vi "DSF.Engine.Plugin.Initialize.vi"(8 "error in (no error)":errorcluster, 10 "Cache":refnum<class "DSF.Engine.Memory.Cache.lvclass">, 11 "Plugin in":refnum<class "DSF.Engine.Plugin.lvclass">) -> (0 "error out":errorcluster, 3 "Plugin out":refnum<class "DSF.Engine.Plugin.lvclass">)   [LabVIEW 2017, in "DSF.Engine.lvlib" / "DSF.Engine.Plugin.lvclass"]
uses:
  DSF.Engine.Plugin.lvclass
  Cache/DSF.Engine.Memory.Cache.lvclass
  DSF.Engine.Plugin.lvclass/DSF.Engine.Plugin.ctl
  Timing/DSF.Engine.Timing.lvclass/DSF.Engine.Timing.ctl
  Debug/DSF.Engine.Debug Flags.lvclass/DSF.Engine.Debug Flags.ctl
  Thread Pool/DSF.Engine.Pool.lvclass/DSF.Engine.Pool.ctl
  Debug/DSF.Engine.Debug Flags.FIFO.lvclass/DSF.Engine.Debug Flags.FIFO.ctl
  Thread Pool/DSF.Engine.Pool.Read FIFO.vi
  Thread Pool/DSF.Engine.Pool.Write FIFO.vi
  Thread Pool/DSF.Engine.Pool.Get FIFO.vi
  Thread Pool/DSF.Engine.Pool.Get Debug Flags.vi
  Debug/DSF.Engine.Debug Flags.FIFO.Get Infinite Timeouts.vi
  Thread Pool/DSF.Engine.Pool.ID.lvclass
  C:/Git/DSF/Source/Engine/Classes/Thread Pool/DSF.Engine.Pool.lvclass
  Transceiver/DSF.Engine.Transceiver Thread.lvclass
  Thread Parameters/Thread Parameters.lvclass
  Timing/DSF.Engine.Timing.lvclass
  Debug/DSF.Engine.Debug Flags.lvclass
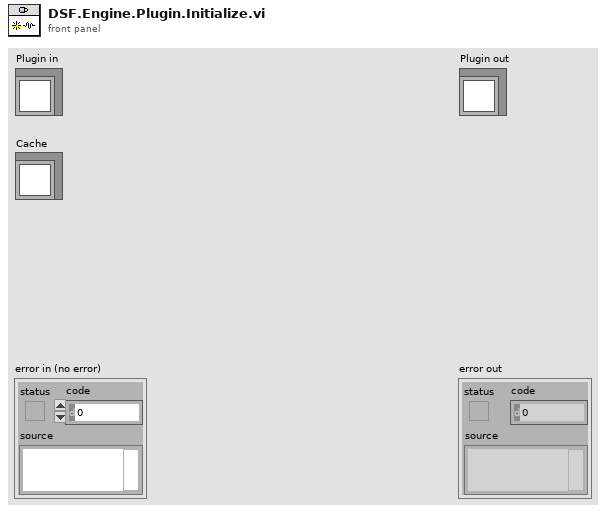
[diagram p1: front panel]
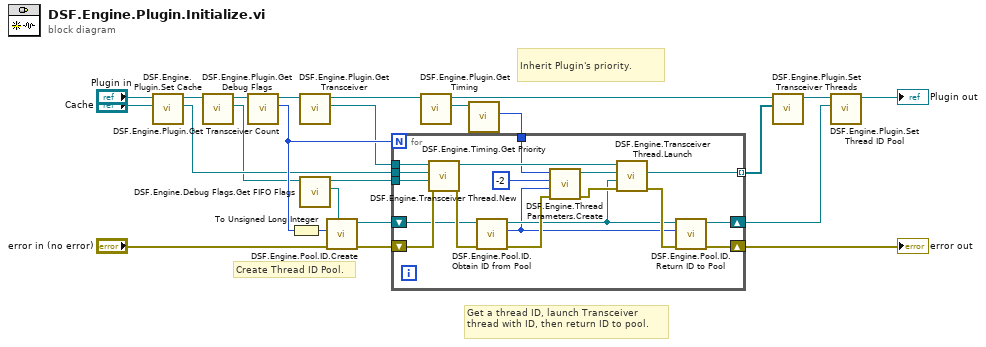
[diagram p0: block diagram]
diagram:
  # "Inherit Plugin's priority."
  # "Get a thread ID, launch Transceiver thread with ID, then return ID to pool."
  # "Create Thread ID Pool."
  n1 = call "DSF.Engine.Plugin.Set Cache.vi"("Cache"="Cache", "Plugin in"="Plugin in") -> ("Plugin out"=w7:refnum<class "DSF.Engine.Plugin.lvclass">)  [unwired: 9 in]
  n2 = call "DSF.Engine.Plugin.Get Debug Flags.vi"("Plugin in"=w7) -> ("Debug Flags"=w4:refnum<class "DSF.Engine.Debug Flags.lvclass">, "Plugin out"=w6:refnum<class "DSF.Engine.Plugin.lvclass">)  [unwired: 9 in]
  n3 = call "DSF.Engine.Plugin.Get Transceiver Count.vi"("Plugin in"=w6) -> ("transceiver count"=w14:i32, "Plugin out"=w19:refnum<class "DSF.Engine.Plugin.lvclass">)  [unwired: 9 in]
  n4 = To Unsigned Long Integer(number=w14) -> (unsigned 32bit integer=w15:u32)
  n5 = call "DSF.Engine.Plugin.Get Transceiver.vi"("Plugin in"=w19) -> ("Transceiver"=w2:refnum<class "DSF.Engine.Transceiver.lvclass">, "Plugin out"=w23:refnum<class "DSF.Engine.Plugin.lvclass">)  [unwired: 9 in]
  n6 = call "DSF.Engine.Debug Flags.Get FIFO Flags.vi"("Debug Flags in"=w4) -> ("FIFO"=w5:refnum<class "DSF.Engine.Debug Flags.FIFO.lvclass">, "Debug Flags out"=w3:refnum<class "DSF.Engine.Debug Flags.lvclass">)  [unwired: 9 in]
  n7 = call "DSF.Engine.Pool.ID.Create.vi"("FIFO Debug Flags"=w5, "error in (no error)"="error in (no error)", "number of IDs"=w15) -> ("error out"=w1:errorcluster, "ID Pool out"=w16:refnum<class "DSF.Engine.Pool.ID.lvclass">)  [unwired: 7 in]
  n8 = call "DSF.Engine.Plugin.Get Timing.vi"("Plugin in"=w23) -> ("Timing"=w18:refnum<class "DSF.Engine.Timing.lvclass">, "Plugin out"=w13:refnum<class "DSF.Engine.Plugin.lvclass">)  [unwired: 9 in]
  n9 = call "DSF.Engine.Timing.Get Priority.vi"("Timing in"=w18) -> ("Priority"=w17:u64)  [unwired: 9 in, 1 out]
  n10 = for {
    N: w14 -> [_]
    tunnel: w2 -> [w41]
    shift-right: [w29] -> w22
    shift-left: w1 -> [w40]
    tunnel: "Cache" -> [w39]
    tunnel: w17 -> [w26]
    tunnel: [w30] -> w12 mode=indexing
    shift-right: [w25] -> w9
    shift-left: w16 -> [w27]
    tunnel: w3 -> [w24]
    n11 = call "DSF.Engine.Transceiver Thread.New.vi"("error in (no error)"=w40, "Debug Flags"=w24, "Cache"=w39, "Transceiver type"=w41) -> ("error out"=w28:errorcluster, "Transceiver Thread out"=w31:refnum<class "DSF.Engine.Transceiver Thread.lvclass">)  [unwired: 6 in]
    n12 = call "DSF.Engine.Pool.ID.Obtain ID from Pool.vi"("error in (no error)"=w28, "ID Pool in"=w27) -> ("error out"=w37:errorcluster, "id"=w32:i32, "ID Pool out"=w34:refnum<class "DSF.Engine.Pool.ID.lvclass">)  [unwired: 6 in, 1 out]
    n13 = call "DSF.Engine.Thread Parameters.Create.vi"("error in (no error)"=w37, "id"=w32, "processor"=-2, "priority"=w26) -> ("error out"=w36:errorcluster, "Thread Parameters"=w33:refnum<class "Thread Parameters.lvclass">)  [unwired: 6 in]
    n14 = call "DSF.Engine.Transceiver Thread.Launch.vi"("error in (no error)"=w36, "Thread ID Pool"=w34, "Thread Parameters"=w33, "Transceiver Thread in"=w31) -> ("error out"=w35:errorcluster, "Interface"=w30:refnum<class "DSF.Engine.Interface.Transceiver.lvclass">)  [unwired: 5 in, 1 out]
    n15 = call "DSF.Engine.Pool.ID.Return ID to Pool.vi"("error in (no error)"=w35, "id"=w32, "ID Pool in"=w34) -> ("error out"=w29:errorcluster, "ID Pool out"=w25:refnum<class "DSF.Engine.Pool.ID.lvclass">)  [unwired: 6 in, 1 out]
  }
  "error out" <- w22
  n16 = call "DSF.Engine.Plugin.Set Transceiver Threads.vi"("Transceiver Threads"=w12, "Plugin in"=w13) -> ("Plugin out"=w11:refnum<class "DSF.Engine.Plugin.lvclass">)  [unwired: 9 in]
  n17 = call "DSF.Engine.Plugin.Set Thread ID Pool.vi"("Thread ID Pool"=w9, "Plugin in"=w11) -> ("Plugin out"=→"Plugin out":refnum<class "DSF.Engine.Plugin.lvclass">)  [unwired: 9 in]
